vi "sincos.vi"() -> ()   [LabVIEW 2015]
uses:
  <vilib>/rvi/FXPMathLib/FxpSinAndCos/subVIs/nifxpmath_SinAndCos_SimConfig.ctl
  <vilib>/Analysis/baseanly.llb/Mean (DBL).vi
  <vilib>/rvi/FXPMathLib/FxpSinAndCos/simVIs/DllFxpSinAndCosTemp_sub.vi
  <vilib>/rvi/FXPMathLib/FxpSinAndCos/XNode/nifxpmath_SinAndCos.xnode
  <vilib>/Analysis/NI_AALBase.lvlib
panel:
  out "cosfxp_mean":dbl format="%0.2f"
  out "sinfxp_mean":dbl format="%0.2f"
  out "cosfxp_max":dbl
  out "sinfxp_max":dbl
  out "stdcosfxp_mean":dbl format="%0.2f"
  out "stdsinfxp_mean":dbl format="%0.2f"
  out "stdcosfxp_max":dbl
  out "stdsinfxp_max":dbl
  out "cossgl_mean":dbl format="%0.2f"
  out "sinsgl_mean":dbl format="%0.2f"
  out "cossgl max":dbl
  out "sinsgl_max":dbl
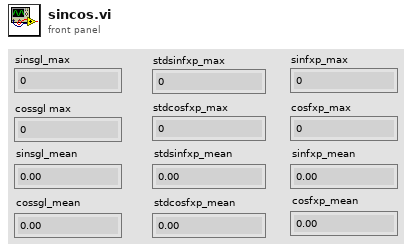
[diagram p1: front panel]
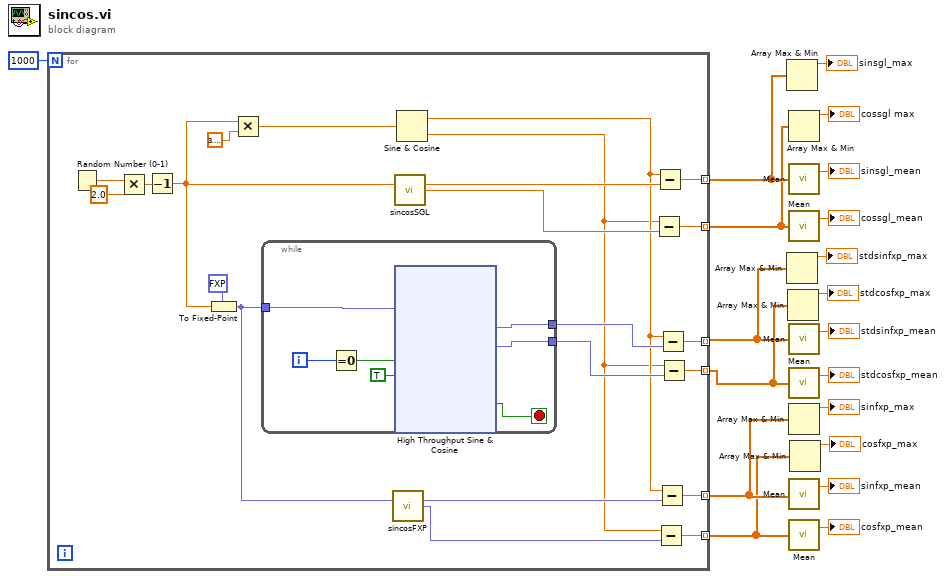
[diagram p0: block diagram]
diagram:
  n1 = for {
    N: 1000 -> [_]
    tunnel: [w29] -> w18 mode=indexing
    tunnel: [w28] -> w17 mode=indexing
    tunnel: [w27] -> w16 mode=indexing
    tunnel: [w26] -> w15 mode=indexing
    tunnel: [w25] -> w14 mode=indexing
    tunnel: [w24] -> w13 mode=indexing
    n2 = Random Number (0-1)() -> (number: 0 to 1=w41:dbl)
    n3 = Multiply(x=w41, y=2.0) -> (x*y=w23:dbl)
    n4 = Decrement(x=w23) -> (x-1=w22:dbl)
    n5 = To Fixed-Point(fixed-point type=fxp<+/-,16,1> 0.0 ("x (pi)"), number=w22) -> (fixed-point=w38:fxp<+/-,16,1>)
    n6 = Multiply(x=w22, y=3.141592653589793) -> (x*y=w21:dbl)
    n7 = while {
      tunnel: w38 -> [w48]
      tunnel: [w43] -> w34
      tunnel: [w42] -> w35
      i -> [w47]
      stop <- w44 stop-if-true
      n8 = Equal To 0?(x=w47) -> (x = 0?=w46:bool)
      n9 = xnode "High Throughput Sine & Cosine"("x (pi)"=w48, "input valid"=w46, "ready for output (T)"=TRUE) -> ("sin(x)"=w43:fxp<+/-,16,2>, "cos(x)"=w42:fxp<+/-,16,2>, "output valid"=w44:bool)  [unwired: 1 out]
    }
    n10 = call "sincosFXP.vi"("x"=w38) -> ("sinx"=w32:fxp<+/-,16,2>, "cosx"=w30:fxp<+/-,16,2>)  [unwired: 13 in]
    n11 = call "sincosSGL.vi"("x"=w22) -> ("sinx"=w37:sgl, "cosx"=w36:sgl)  [unwired: 13 in]
    n12 = Sine & Cosine(0:w21) -> (1:w33:dbl, 2:w31:dbl)
    n13 = Subtract(x=w31, y=w36) -> (x-y=w28:dbl)
    n14 = Subtract(x=w33, y=w37) -> (x-y=w29:dbl)
    n15 = Subtract(x=w31, y=w30) -> (x-y=w24:dbl)
    n16 = Subtract(x=w33, y=w32) -> (x-y=w25:dbl)
    n17 = Subtract(x=w33, y=w34) -> (x-y=w27:dbl)
    n18 = Subtract(x=w31, y=w35) -> (x-y=w26:dbl)
  }
  n19 = Array Max & Min(array=w18) -> (max value=→"sinsgl_max":dbl)  [unwired: 3 out]
  n20 = Array Max & Min(array=w16) -> (max value=→"stdsinfxp_max":dbl)  [unwired: 3 out]
  n21 = Array Max & Min(array=w15) -> (max value=→"stdcosfxp_max":dbl)  [unwired: 3 out]
  n22 = Array Max & Min(array=w17) -> (max value=→"cossgl max":dbl)  [unwired: 3 out]
  n23 = call-poly <vilib>:"Mean.vi"("X"=w18) -> ("mean"=→"sinsgl_mean":dbl)  [unwired: 1 out]
  n24 = call-poly <vilib>:"Mean.vi"("X"=w17) -> ("mean"=→"cossgl_mean":dbl)  [unwired: 1 out]
  n25 = call-poly <vilib>:"Mean.vi"("X"=w16) -> ("mean"=→"stdsinfxp_mean":dbl)  [unwired: 1 out]
  n26 = call-poly <vilib>:"Mean.vi"("X"=w15) -> ("mean"=→"stdcosfxp_mean":dbl)  [unwired: 1 out]
  n27 = Array Max & Min(array=w14) -> (max value=→"sinfxp_max":dbl)  [unwired: 3 out]
  n28 = call-poly <vilib>:"Mean.vi"("X"=w14) -> ("mean"=→"sinfxp_mean":dbl)  [unwired: 1 out]
  n29 = call-poly <vilib>:"Mean.vi"("X"=w13) -> ("mean"=→"cosfxp_mean":dbl)  [unwired: 1 out]
  n30 = Array Max & Min(array=w13) -> (max value=→"cosfxp_max":dbl)  [unwired: 3 out]
